vi "Raster_2DOutput_wCounter_82_EXP.vi"(2 "Save File path":path, 3 "Save?":bool=TRUE, 6 "error in":errorcluster, 7 "Update Rate (Hz)":dbl=100.0, 8 "Y Parameters":T1={"Number of Y Steps"=200, "Max Y (V)"=2.0, "Min Y (V)"=-2.0}, 9 "X Parameters":T2={"Number of X Steps"=200, "Max X (V)"=2.0, "Min X (V)"=-2.0}) -> (0 "error out":errorcluster, 1 "Intensity Graph":dbl[][](graph))   [LabVIEW 2011]
uses:
  <vilib>/DAQmx/write.llb/DAQmx Write (Analog 2D DBL NChan NSamp).vi
  <vilib>/DAQmx/read.llb/DAQmx Read (Counter 1D U32 1Chan NSamp).vi
  <vilib>/DAQmx/create/channels.llb/DAQmx Create Channel (CI-Count Edges).vi
  <vilib>/DAQmx/configure/timing.llb/DAQmx Timing (Sample Clock).vi
  <vilib>/DAQmx/create/channels.llb/DAQmx Create Channel (AO-Voltage-Basic).vi
  <vilib>/DAQmx/miscellaneous.llb/DAQmx Fill In Error Info.vi
  Program Files/National Instruments/LabVIEW 2011/resource/objmgr/daqmx.rc
panel:
  out "TotalSampPerChanAcquired":dbl
  out "Output:":dbl[][](graph)
  in  "stop":bool
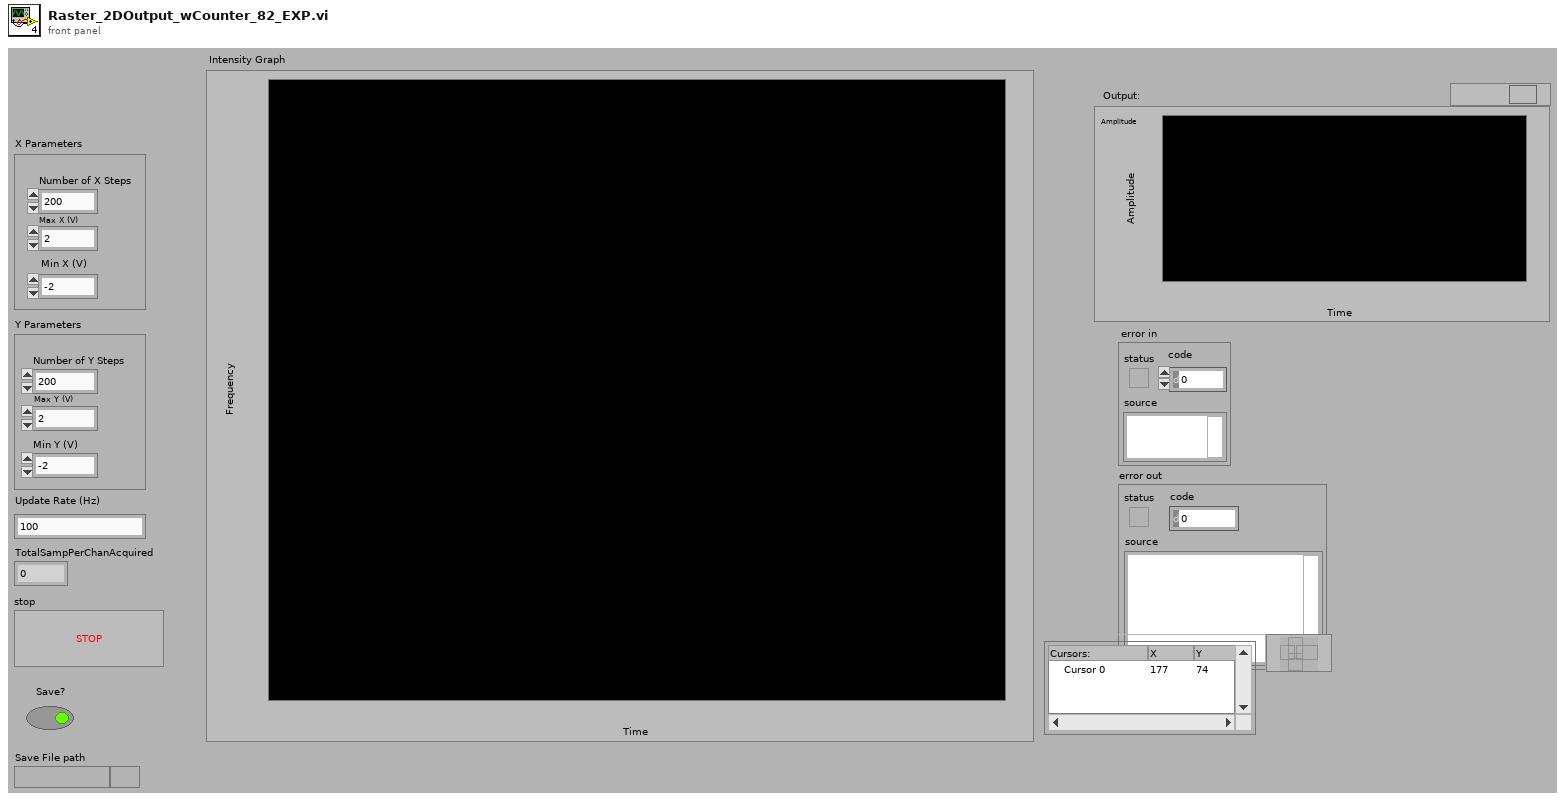
[diagram p1: front panel]
types:
  T1 = cluster{"Number of Y Steps":i32, "Max Y (V)":dbl, "Min Y (V)":dbl}
  T2 = cluster{"Number of X Steps":i32, "Max X (V)":dbl, "Min X (V)":dbl}
  T3 = typedef "imagedata.ctl" = cluster{"image type":i32, "image depth":i32, "image":u8[], "mask":u8[], "colors":u32[], "Rectangle":cluster{"left":i16, "top":i16, "right":i16, "bottom":i16}}
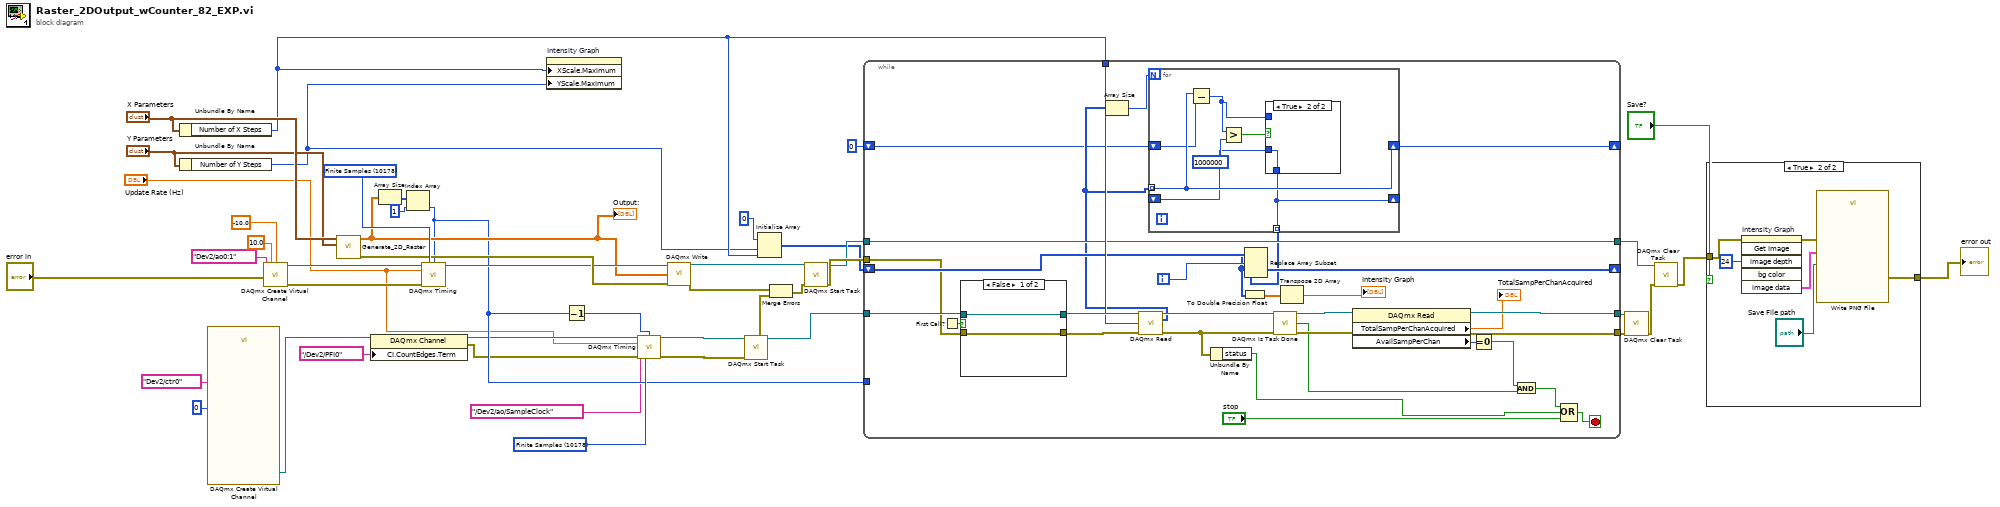
[diagram p0: block diagram]
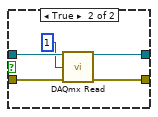
[diagram p4: hidden frame]
diagram:
  w37 = 10178 items=["Finite Samples"=10178, "Continuous Samples"=10123, "Hardware Timed Single Point"=12522] ("sample mode")
  w38 = 10178 items=["Finite Samples"=10178, "Continuous Samples"=10123, "Hardware Timed Single Point"=12522] ("sample mode")
  n1 = Unbundle By Name("X Parameters") -> ("Number of X Steps"=w2:i32)
  n2 = Unbundle By Name("Y Parameters") -> ("Number of Y Steps"=w1:i32)
  n3 = call-poly <vilib>:"DAQmx Create Virtual Channel.vi"("initial count"=u32 0, "counter"=tag "Dev2/ctr0") -> ("task out"=w12:refnum<k21>)  [unwired: 6 in, 7 out]
  n4 = call-poly <vilib>:"DAQmx Create Virtual Channel.vi"("maximum value"=10.0, "minimum value"=-10.0, "physical channels"=tag "Dev2/ao0:1", "error in"="error in") -> ("task out"=w46:refnum<k21>, "error out"=w45:errorcluster)  [unwired: 5 in, 5 out]
  n5 = call "Generate_2D_Raster.vi"("Y Parameters"="Y Parameters", "X Parameters"="X Parameters") -> ("error IO"=w29:errorcluster, "Array"=w23:dbl[][])  [unwired: 1 in, 7 out]
  "Output:" <- w23
  n6 = property class="DAQmx Channel"(reference=w12, "CI.CountEdges.Term"=tag "/Dev2/PFI0") -> (reference out=w11:refnum<k21>, error out=w8:errorcluster)  [unwired: 1 in]
  n7 = Array Size(array=w23) -> (size(s)=w22:i32[])
  n8 = Index Array(array=w22, index=1) -> (element=w20:i32)
  n9 = call-poly <vilib>:"DAQmx Timing.vi"("task/channels in"=w46, "sample mode"=w38, "samples per channel"=w20, "rate"="Update Rate (Hz)", "error in"=w45) -> ("task out"=w24:refnum<k21>)  [unwired: 2 in, 8 out]
  n10 = property on="Intensity Graph" class="IntGraph (strict)"("XScale.Maximum"=w2, "YScale.Maximum"=w1) -> ()  [unwired: 2 in, 2 out]
  n11 = Decrement(x=w20) -> (x-1=w17:i32)
  n12 = call-poly <vilib>:"DAQmx Timing.vi"("task/channels in"=w11, "sample mode"=w37, "samples per channel"=w17, "rate"="Update Rate (Hz)", "source"=tag "/Dev2/ao/SampleClock", "error in"=w8) -> ("task out"=w43:refnum<k21>, "error out"=w3:errorcluster)  [unwired: 1 in, 7 out]
  n13 = call-poly <vilib>:"DAQmx Write.vi"("task/channels in"=w24, "data"=w23, "error in"=w29) -> ("task out"=w42:refnum<k21>, "error out"=w31:errorcluster)  [unwired: 1 in, 10 out]
  n14 = call <vilib>:"DAQmx Start Task.vi"("task/channels in"=w43, "error in"=w3) -> ("task out"=w39:refnum<k21>, "error out"=w30:errorcluster)  [unwired: 12 out]
  n15 = Initialize Array(u32 0, w1, w2) -> (w25:u32[][])
  n16 = Merge Errors(w31, w30) -> (w32:errorcluster)
  n17 = call <vilib>:"DAQmx Start Task.vi"("task/channels in"=w42, "error in"=w32) -> ("task out"=w40:refnum<k21>, "error out"=w41:errorcluster)  [unwired: 12 out]
  n18 = while {
    tunnel: w40 -> [w67]
    tunnel: w41 -> [w68]
    tunnel: w39 -> [w76]
    tunnel: [w67] -> w36
    tunnel: w2 -> [w72]
    shift-right: [w69] -> _
    shift-left: w25 -> [w71]
    tunnel: w20 -> [_]
    tunnel: [w63] -> w19
    tunnel: [w64] -> w18
    shift-right: [w49] -> _
    shift-left: u32 0 ("Numeric") -> [w48]
    i -> [w70]
    stop <- w77 stop-if-true
    n19 = First Call?() -> (First Call?: T/F=w73:bool)
    n20 = case shown="False" w73 {
      tunnel: w76 -> [w88 w93]
      tunnel: [w88 w92] -> w75
      tunnel: [w87 w91] -> w74
      tunnel: w68 -> [w87 w90]
      frame False {
      }
      frame True {
        n21 = call-poly <vilib>:"DAQmx Read.vi"("task/channels in"=w93, "number of samples per channel"=1, "error in"=w90) -> ("task out"=w92:refnum<k21>, "error out"=w91:errorcluster)  [unwired: 11 out]
      }
    }
    n22 = call-poly <vilib>:"DAQmx Read.vi"("task/channels in"=w75, "number of samples per channel"=w72, "error in"=w74) -> ("task out"=w65:refnum<k21>, "data"=w51:u32[], "error out"=w56:errorcluster)  [unwired: 1 in, 9 out]
    n23 = Array Size(array=w51) -> (size(s)=w52:i32)
    n24 = for {
      N: w52 -> [_]
      tunnel: w51 -> [w84] mode=indexing
      shift-right: [w84] -> w49
      shift-left: w48 -> [w83]
      tunnel: [w79] -> w50 mode=indexing
      shift-right: [w79] -> _
      shift-left: _ -> [w78]
      n25 = Subtract(x=w84, y=w83) -> (x-y=w80:u32)
      n26 = Greater?(x=w80, y=u32 1000000) -> (0:w81:bool)
      n27 = case shown="True" w81 {
        tunnel: w80 -> [w85 _]
        tunnel: [w85 w86] -> w79
        tunnel: w78 -> [_ w86]
        frame False {
        }
        frame True {
        }
      }
    }
    n28 = Unbundle By Name(w56) -> ("status"=w54:bool)
    n29 = Replace Array Subset(array=w71, new element=w50, index (row)=w70) -> (w69:u32[][])  [unwired: 1 in]
    n30 = To Double Precision Float(number=w69) -> (double precision float=w66:dbl[][])
    n31 = call <vilib>:"DAQmx Is Task Done.vi"("task/channels in"=w65, "error in"=w56) -> ("task out"=w62:refnum<k21>, "task done?"=w59:bool, "error out"=w61:errorcluster)  [unwired: 11 out]
    n32 = Transpose 2D Array(2D array=w66) -> (transposed array=→"Intensity Graph":dbl[][])
    n33 = property class="DAQmx Read"(reference=w62, error in=w61) -> (reference out=w64:refnum<k21>, error out=w63:errorcluster, "TotalSampPerChanAcquired"=→"TotalSampPerChanAcquired":dbl, "AvailSampPerChan"=w58:u32)
    n34 = Equal To 0?(x=w58) -> (x = 0?=w57:bool)
    n35 = And(x=w57, y=w59) -> (x .and. y?=w53:bool)
    n36 = Compound Arithmetic op=OR(w53, w54, "stop") -> (w77:bool)
  }
  n37 = call <vilib>:"DAQmx Clear Task.vi"("task in"=w18, "error in"=w19) -> ("error out"=w33:errorcluster)  [unwired: 13 out]
  n38 = call <vilib>:"DAQmx Clear Task.vi"("task in"=w36, "error in"=w33) -> ("error out"=w16:errorcluster)  [unwired: 13 out]
  n39 = case shown="True" "Save?" {
    tunnel: w16 -> [w94 w98]
    tunnel: [w94 w100] -> w15
    frame False {
    }
    frame True {
      n40 = invoke on="Intensity Graph" class="IntGraph (strict)" method="Get Image"(error in=w98, "image depth"=24 ("Image Depth")) -> (error out=w97:errorcluster, "image data"=w96:T3)  [unwired: 4 in, 4 out]
      n41 = call <vilib>:"Write PNG File.vi"("error in (no error)"=w97, "image data"=w96, "path to PNG file"="Save File path") -> ("error out"=w100:errorcluster)  [unwired: 7 in, 1 out]
    }
  }
  "error out" <- w15
